vi "ReceiveData.vi"(0 "设备类型":u32(ring)=3 items=["PCI5121"=1, "PCI9810"=2, "USBCAN1"=3, "USBCAN2"=4, "PCI9820"=5, "PCI5110"=7, "PC104CAN"=11, "CANETUDP"=12, "PCI9840B"=14, "PC104C2"=15, "PCI9820I"=16, "CANETTCP"=17, "PCIE9221"=24], 5 "索引号":u32, 7 "CAN通道":u32, 9 "arraylen":u32=1, 11 "错误输入":errorcluster caption="错误输入（无错误）", 12 "TimeOut":i32=150) -> (4 "DeviceType":u32, 6 "VCI_CAN_OBJ_RN":T1(array[cluster]) {"Byte7" format="%02x"; "Byte6" format="%02x"; "Byte5" format="%02x"; "Byte4" format="%02x"; "Byte3" format="%02x"; "Byte2" format="%02x"; "Byte1" format="%02x"; "Byte0" format="%02x"; "ID" format="%02x"}, 8 "Result":bool, 10 "Len":u32, 15 "错误输出":errorcluster)   [LabVIEW 2013]
uses:
  GlobalVariable.vi
  ControlCAN.dll
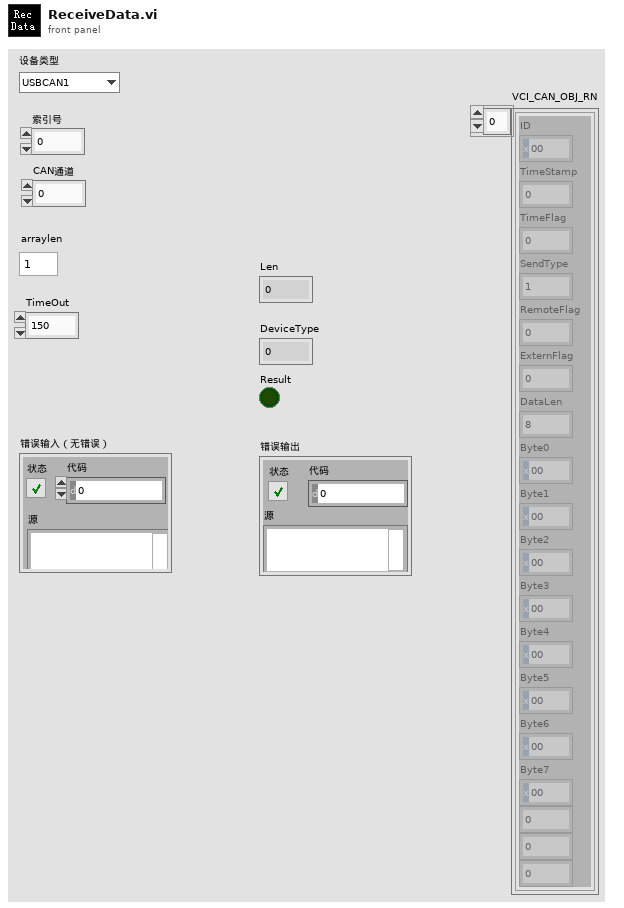
[diagram p1: front panel]
types:
  T1 = cluster{"ID":u32, "TimeStamp":u32, "TimeFlag":u8, "SendType":u8, "RemoteFlag":u8, "ExternFlag":u8, "DataLen":u8, "Byte0":u8, "Byte1":u8, "Byte2":u8, "Byte3":u8, "Byte4":u8, "Byte5":u8, "Byte6":u8, "Byte7":u8, u8, u8, u8}[]
  T2 = cluster{"ID":u32, "TimeStamp":u32, "TimeFlag":u8, "SendType":u8, "RemoteFlag":u8, "ExternFlag":u8, "DataLen":u8, u8, u8, u8, u8, u8, u8, u8, u8, u8, u8, u8}[]
  T3 = cluster{"ID":u32, "TimeStamp":u32, "TimeFlag":u8, "SendType":u8, "RemoteFlag":u8, "ExternFlag":u8, "DataLen":u8, u8, u8, u8, u8, u8, u8, u8, u8, u8, u8, u8}
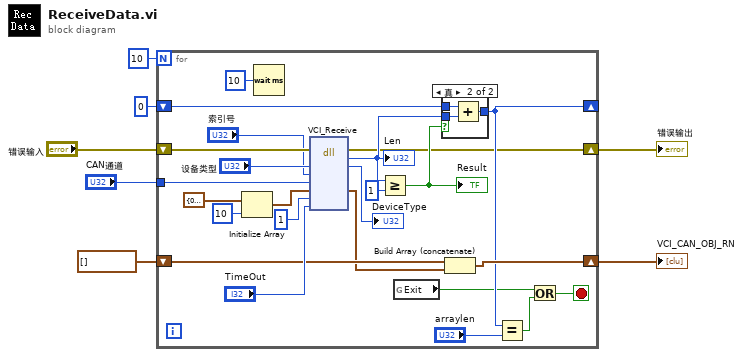
[diagram p0: block diagram]
diagram:
  n1 = for {
    N: 10 -> [_]
    shift-right: [w23] -> w4
    shift-left: T2 [] -> [w25]
    shift-right: [w18] -> _
    shift-left: u32 0 -> [w22]
    shift-right: [w14] -> w3
    shift-left: "错误输入" -> [w13]
    tunnel: "CAN通道" -> [w8]
    stop <- w10 stop-if-true
    n2 = Initialize Array(T3 {"ID"=0, "TimeStamp"=0, "TimeFlag"=0, "SendType"=1, "RemoteFlag"=0, "ExternFlag"=0, "DataLen"=8, 0, 0, 0, 0, 0, 0, 0, 0, 0, 0, 0} ("VCI_CAN_OBJ_R"), 10 ("维数大小")) -> (w28:T2)
    n3 = Wait (ms)(milliseconds to wait=u32 10 ("等待时间（毫秒）")) -> ()  [unwired: 1 out]
    n4 = dll-call lib="PTH1Aabs F吉利吉利CAN模拟器CAN_ZLGCANControlCAN.dll" fn="VCI_Receive"(error in=w13, "DeviceType"="设备类型", "DeviceInd"="索引号", "CANInd"=w8, "pReceive"=w28, "Len"=u32 1, "WaitTime"="TimeOut") -> (error out=w14:errorcluster, "return type"=w21:u32, "DeviceType"=→"DeviceType":u32, "pReceive"=w24:T2)  [unwired: 6 in, 1 out]
    "Len" <- w21
    n5 = Greater Or Equal?(x=w21, y=u32 1) -> (x >= y?=w20:bool)
    "Result" <- w20
    n6 = global read "GlobalVariable.vi" "Exit"() -> (w12:bool)
    n7 = case shown="真" w20 {
      tunnel: w21 -> [_ w35]
      tunnel: w22 -> [w32 w34]
      tunnel: [w32 w33] -> w18
      frame False {
      }
      frame True {
        n8 = Add(x=w34, y=w35) -> (x+y=w33:u32)
      }
    }
    n9 = Build Array (concatenate)(w25, w24) -> (w23:T2)
    n10 = Equal?(x=w18, y="arraylen") -> (x = y?=w11:bool)
    n11 = Or(x=w12, y=w11) -> (x .or. y?=w10:bool)
  }
  "VCI_CAN_OBJ_RN" <- w4
  "错误输出" <- w3
